vi "BitwiseORGreyscale.vi"(8 "error in (no error)":errorcluster, 9 "Greyscale Image Destination":refnum<data-value>, 10 "Greyscale Image B":refnum<data-value>, 11 "Greyscale Image A":refnum<data-value>) -> (0 "error out":errorcluster, 3 "Greyscale Image Destination (duplicate)":refnum<data-value>)   [LabVIEW 2020, in "g_ar_toolkit.image.lvlib"]
uses:
  g_ar_toolkit.image.lvlib
  BitwiseOperation.ctl
  <vilib>/Utility/error.llb/Error Cluster From Error Code.vi
  0e84d7da-7af3-4d73-801a-9d94e7981347.vi
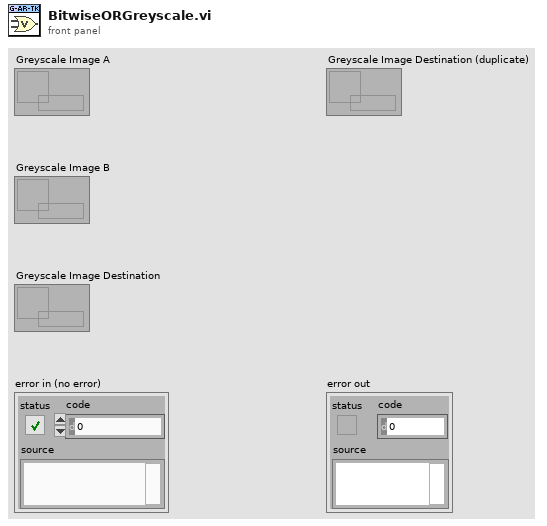
[diagram p1: front panel]
types:
  T1 = typedef "g_ar_toolkit.image.lvlib/BitwiseOperation.ctl" = enum8{"OR", "AND", "XOR"}
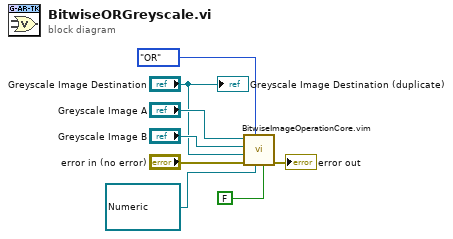
[diagram p0: block diagram]
diagram:
  n1 = call "BitwiseImageOperationCore.vim"("HasMask"=FALSE, "Mask"=refnum<data-value> refnum, "BitwiseOperation"=BitwiseOperation."OR", "error in (no error)"="error in (no error)", "Destination Image"="Greyscale Image Destination", "Image B"="Greyscale Image B", "Image A"="Greyscale Image A") -> ("error out"=→"error out":errorcluster)  [unwired: 4 in]
  "Greyscale Image Destination (duplicate)" <- "Greyscale Image Destination"
